vi "MotionProfileGeneratorFilter2Sum.vi"(2 "Filter Queue":refnum<queue>, 3 "Filter1Sum":dbl) -> (0 "queue out":refnum<queue>, 1 "Filter2Sum":dbl)   [LabVIEW 2018, in "ArgosLib.lvlib"]
uses:
  ArgosLib.lvlib
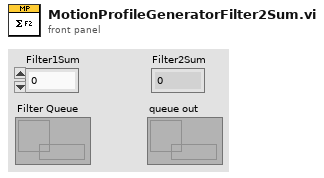
[diagram p1: front panel]
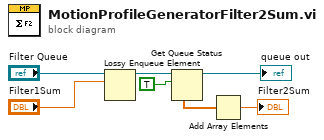
[diagram p0: block diagram]
diagram:
  n1 = Lossy Enqueue Element(queue="Filter Queue", element="Filter1Sum") -> (queue out=w7:refnum<queue>)  [unwired: 1 in, 3 out]
  n2 = Get Queue Status(queue=w7, return elements? (F)=TRUE) -> (queue out=→"queue out":refnum<queue>, elements=w5:dbl[])  [unwired: 1 in, 6 out]
  n3 = Add Array Elements(numeric array=w5) -> (sum=→"Filter2Sum":dbl)
